vi "generate_plot.vi"(6 "High Voltage":sgl=2.0, 7 "Sens":dbl=12100000000000.0, 10 "Vnoise":dbl=0.005, 11 "Dust Array":T2[](array[typedef])=[{"Dust Event ID"=59, "Integer Timestamp"=1340138392671, "Velocity"=19145.19921875, "Mass"=9.709090342484041e-18, "Charge"=8.89689e-16, "Radius"=6.65219e-08, "Passed_3rd_Detector"=1, "High Voltage"=2.0, "+ High Voltage Supply"=0.0, "- High Voltage Supply"=0.0, "HV Control Difference"=0.0, "Vacuum Pressure"=0.0, "Radiation"=0.0, "Column Current"=0.0, "Lost Charge"=0.0, "Chain Current"=0.0, "Control High Voltage"=0.0, "Current Group Name:"="New Group Name", "Current Experiment Name:"="test", "Current Experiment Description:"="", "Estimate Source"=1, "Estimate Quality"=1, "File Location"=0, "Dust Type"="", "Dust Density"=0.0}, {"Dust Event ID"=61, "Integer Timestamp"=1340138406852, "Velocity"=9417.3203125, "Mass"=5.304340014877123e-17, "Charge"=1.17605e-15, "Radius"=1.17161e-07, "Passed_3rd_Detector"=1, "High Voltage"=2.0, "+ High Voltage Supply"=0.0, "- High Voltage Supply"=0.0, "HV Control Difference"=0.0, "Vacuum Pressure"=0.0, "Radiation"=0.0, "Column Current"=0.0, "Lost Charge"=0.0, "Chain Current"=0.0, "Control High Voltage"=0.0, "Current Group Name:"="New Group Name", "Current Experiment Name:"="test", "Current Experiment Description:"="", "Estimate Source"=1, "Estimate Quality"=1, "File Location"=0, "Dust Type"="", "Dust Density"=0.0}, {"Dust Event ID"=63, "Integer Timestamp"=1340138434737, "Velocity"=6076.06982421875, "Mass"=5.564189870760041e-17, "Charge"=5.13556e-16, "Radius"=1.19044e-07, "Passed_3rd_Detector"=1, "High Voltage"=2.0, "+ High Voltage Supply"=0.0, "- High Voltage Supply"=0.0, "HV Control Difference"=0.0, "Vacuum Pressure"=0.0, "Radiation"=0.0, "Column Current"=0.0, "Lost Charge"=0.0, "Chain Current"=0.0, "Control High Voltage"=0.0, "Current Group Name:"="New Group Name", "Current Experiment Name:"="test", "Current Experiment Description:"="", "Estimate Source"=1, "Estimate Quality"=1, "File Location"=0, "Dust Type"="", "Dust Density"=0.0}, {"Dust Event ID"=65, "Integer Timestamp"=1340138517545, "Velocity"=5796.47021484375, "Mass"=7.827660164472748e-16, "Charge"=6.57505e-15, "Radius"=2.87375e-07, "Passed_3rd_Detector"=1, "High Voltage"=2.0, "+ High Voltage Supply"=0.0, "- High Voltage Supply"=0.0, "HV Control Difference"=0.0, "Vacuum Pressure"=0.0, "Radiation"=0.0, "Column Current"=0.0, "Lost Charge"=0.0, "Chain Current"=0.0, "Control High Voltage"=0.0, "Current Group Name:"="New Group Name", "Current Experiment Name:"="test", "Current Experiment Description:"="", "Estimate Source"=1, "Estimate Quality"=1, "File Location"=0, "Dust Type"="", "Dust Density"=0.0}, {"Dust Event ID"=66, "Integer Timestamp"=1340138518480, "Velocity"=9192.0595703125, "Mass"=9.891599803709986e-17, "Charge"=2.08945e-15, "Radius"=1.4421e-07, "Passed_3rd_Detector"=1, "High Voltage"=2.0, "+ High Voltage Supply"=0.0, "- High Voltage Supply"=0.0, "HV Control Difference"=0.0, "Vacuum Pressure"=0.0, "Radiation"=0.0, "Column Current"=0.0, "Lost Charge"=0.0, "Chain Current"=0.0, "Control High Voltage"=0.0, "Current Group Name:"="New Group Name", "Current Experiment Name:"="test", "Current Experiment Description:"="", "Estimate Source"=1, "Estimate Quality"=1, "File Location"=0, "Dust Type"="", "Dust Density"=0.0}, {"Dust Event ID"=67, "Integer Timestamp"=1340138532228, "Velocity"=34719.30078125, "Mass"=2.6360200918000455e-18, "Charge"=7.94385e-16, "Radius"=4.30746e-08, "Passed_3rd_Detector"=1, "High Voltage"=2.0, "+ High Voltage Supply"=0.0, "- High Voltage Supply"=0.0, "HV Control Difference"=0.0, "Vacuum Pressure"=0.0, "Radiation"=0.0, "Column Current"=0.0, "Lost Charge"=0.0, "Chain Current"=0.0, "Control High Voltage"=0.0, "Current Group Name:"="New Group Name", "Current Experiment Name:"="test", "Current Experiment Description:"="", "Estimate Source"=1, "Estimate Quality"=1, "File Location"=0, "Dust Type"="", "Dust Density"=0.0}, {"Dust Event ID"=68, "Integer Timestamp"=1340138545545, "Velocity"=7001.97021484375, "Mass"=1.8855600591991987e-16, "Charge"=2.31111e-15, "Radius"=1.78807e-07, "Passed_3rd_Detector"=1, "High Voltage"=2.0, "+ High Voltage Supply"=0.0, "- High Voltage Supply"=0.0, "HV Control Difference"=0.0, "Vacuum Pressure"=0.0, "Radiation"=0.0, "Column Current"=0.0, "Lost Charge"=0.0, "Chain Current"=0.0, "Control High Voltage"=0.0, "Current Group Name:"="New Group Name", "Current Experiment Name:"="test", "Current Experiment Description:"="", "Estimate Source"=1, "Estimate Quality"=1, "File Location"=0, "Dust Type"="", "Dust Density"=0.0}, {"Dust Event ID"=73, "Integer Timestamp"=1340138752578, "Velocity"=19658.5, "Mass"=9.036869609983635e-18, "Charge"=8.7309e-16, "Radius"=6.49498e-08, "Passed_3rd_Detector"=1, "High Voltage"=2.0, "+ High Voltage Supply"=0.0, "- High Voltage Supply"=0.0, "HV Control Difference"=0.0, "Vacuum Pressure"=0.0, "Radiation"=0.0, "Column Current"=0.0, "Lost Charge"=0.0, "Chain Current"=0.0, "Control High Voltage"=0.0, "Current Group Name:"="New Group Name", "Current Experiment Name:"="test", "Current Experiment Description:"="", "Estimate Source"=1, "Estimate Quality"=1, "File Location"=0, "Dust Type"="", "Dust Density"=0.0}, {"Dust Event ID"=74, "Integer Timestamp"=1340138757697, "Velocity"=26103.69921875, "Mass"=5.479880065852002e-18, "Charge"=9.33502e-16, "Radius"=5.49746e-08, "Passed_3rd_Detector"=1, "High Voltage"=2.0, "+ High Voltage Supply"=0.0, "- High Voltage Supply"=0.0, "HV Control Difference"=0.0, "Vacuum Pressure"=0.0, "Radiation"=0.0, "Column Current"=0.0, "Lost Charge"=0.0, "Chain Current"=0.0, "Control High Voltage"=0.0, "Current Group Name:"="New Group Name", "Current Experiment Name:"="test", "Current Experiment Description:"="", "Estimate Source"=1, "Estimate Quality"=1, "File Location"=0, "Dust Type"="", "Dust Density"=0.0}, {"Dust Event ID"=75, "Integer Timestamp"=1340138762289, "Velocity"=11104.599609375, "Mass"=3.4991500151336583e-17, "Charge"=1.07872e-15, "Radius"=1.0199e-07, "Passed_3rd_Detector"=1, "High Voltage"=2.0, "+ High Voltage Supply"=0.0, "- High Voltage Supply"=0.0, "HV Control Difference"=0.0, "Vacuum Pressure"=0.0, "Radiation"=0.0, "Column Current"=0.0, "Lost Charge"=0.0, "Chain Current"=0.0, "Control High Voltage"=0.0, "Current Group Name:"="New Group Name", "Current Experiment Name:"="test", "Current Experiment Description:"="", "Estimate Source"=1, "Estimate Quality"=1, "File Location"=0, "Dust Type"="", "Dust Density"=0.0}, {"Dust Event ID"=76, "Integer Timestamp"=1340138792956, "Velocity"=7613.759765625, "Mass"=1.7990099679509583e-16, "Charge"=2.60719e-15, "Radius"=1.76029e-07, "Passed_3rd_Detector"=1, "High Voltage"=2.0, "+ High Voltage Supply"=0.0, "- High Voltage Supply"=0.0, "HV Control Difference"=0.0, "Vacuum Pressure"=0.0, "Radiation"=0.0, "Column Current"=0.0, "Lost Charge"=0.0, "Chain Current"=0.0, "Control High Voltage"=0.0, "Current Group Name:"="New Group Name", "Current Experiment Name:"="test", "Current Experiment Description:"="", "Estimate Source"=1, "Estimate Quality"=1, "File Location"=0, "Dust Type"="", "Dust Density"=0.0}, {"Dust Event ID"=80, "Integer Timestamp"=1340139107484, "Velocity"=34660.0, "Mass"=2.9206500454473984e-18, "Charge"=8.77155e-16, "Radius"=4.45723e-08, "Passed_3rd_Detector"=1, "High Voltage"=2.0, "+ High Voltage Supply"=0.0, "- High Voltage Supply"=0.0, "HV Control Difference"=0.0, "Vacuum Pressure"=0.0, "Radiation"=0.0, "Column Current"=0.0, "Lost Charge"=0.0, "Chain Current"=0.0, "Control High Voltage"=0.0, "Current Group Name:"="New Group Name", "Current Experiment Name:"="test", "Current Experiment Description:"="", "Estimate Source"=1, "Estimate Quality"=1, "File Location"=0, "Dust Type"="", "Dust Density"=0.0}, {"Dust Event ID"=85, "Integer Timestamp"=1340139269076, "Velocity"=7758.72021484375, "Mass"=1.2614399785804245e-16, "Charge"=1.89839e-15, "Radius"=1.56385e-07, "Passed_3rd_Detector"=1, "High Voltage"=2.0, "+ High Voltage Supply"=0.0, "- High Voltage Supply"=0.0, "HV Control Difference"=0.0, "Vacuum Pressure"=0.0, "Radiation"=0.0, "Column Current"=0.0, "Lost Charge"=0.0, "Chain Current"=0.0, "Control High Voltage"=0.0, "Current Group Name:"="New Group Name", "Current Experiment Name:"="test", "Current Experiment Description:"="", "Estimate Source"=1, "Estimate Quality"=1, "File Location"=0, "Dust Type"="", "Dust Density"=0.0}, {"Dust Event ID"=90, "Integer Timestamp"=1340139421851, "Velocity"=7551.02001953125, "Mass"=1.7357100046625623e-16, "Charge"=2.47417e-15, "Radius"=1.73939e-07, "Passed_3rd_Detector"=1, "High Voltage"=2.0, "+ High Voltage Supply"=0.0, "- High Voltage Supply"=0.0, "HV Control Difference"=0.0, "Vacuum Pressure"=0.0, "Radiation"=0.0, "Column Current"=0.0, "Lost Charge"=0.0, "Chain Current"=0.0, "Control High Voltage"=0.0, "Current Group Name:"="New Group Name", "Current Experiment Name:"="test", "Current Experiment Description:"="", "Estimate Source"=1, "Estimate Quality"=1, "File Location"=0, "Dust Type"="", "Dust Density"=0.0}, {"Dust Event ID"=92, "Integer Timestamp"=1340139600351, "Velocity"=17512.5, "Mass"=1.0332900329634781e-17, "Charge"=7.9224e-16, "Radius"=6.7917e-08, "Passed_3rd_Detector"=1, "High Voltage"=2.0, "+ High Voltage Supply"=0.0, "- High Voltage Supply"=0.0, "HV Control Difference"=0.0, "Vacuum Pressure"=0.0, "Radiation"=0.0, "Column Current"=0.0, "Lost Charge"=0.0, "Chain Current"=0.0, "Control High Voltage"=0.0, "Current Group Name:"="New Group Name", "Current Experiment Name:"="test", "Current Experiment Description:"="", "Estimate Source"=1, "Estimate Quality"=1, "File Location"=0, "Dust Type"="", "Dust Density"=0.0}, {"Dust Event ID"=95, "Integer Timestamp"=1340139724238, "Velocity"=28180.69921875, "Mass"=4.071129857718561e-18, "Charge"=8.08274e-16, "Radius"=4.97902e-08, "Passed_3rd_Detector"=1, "High Voltage"=2.0, "+ High Voltage Supply"=0.0, "- High Voltage Supply"=0.0, "HV Control Difference"=0.0, "Vacuum Pressure"=0.0, "Radiation"=0.0, "Column Current"=0.0, "Lost Charge"=0.0, "Chain Current"=0.0, "Control High Voltage"=0.0, "Current Group Name:"="New Group Name", "Current Experiment Name:"="test", "Current Experiment Description:"="", "Estimate Source"=1, "Estimate Quality"=1, "File Location"=0, "Dust Type"="", "Dust Density"=0.0}, {"Dust Event ID"=97, "Integer Timestamp"=1340139740652, "Velocity"=7861.9599609375, "Mass"=5.145899855115246e-17, "Charge"=7.95176e-16, "Radius"=1.15983e-07, "Passed_3rd_Detector"=1, "High Voltage"=2.0, "+ High Voltage Supply"=0.0, "- High Voltage Supply"=0.0, "HV Control Difference"=0.0, "Vacuum Pressure"=0.0, "Radiation"=0.0, "Column Current"=0.0, "Lost Charge"=0.0, "Chain Current"=0.0, "Control High Voltage"=0.0, "Current Group Name:"="New Group Name", "Current Experiment Name:"="test", "Current Experiment Description:"="", "Estimate Source"=1, "Estimate Quality"=1, "File Location"=0, "Dust Type"="", "Dust Density"=0.0}, {"Dust Event ID"=105, "Integer Timestamp"=1340140151192, "Velocity"=6723.72021484375, "Mass"=2.712949915359978e-16, "Charge"=3.0662e-15, "Radius"=2.01861e-07, "Passed_3rd_Detector"=1, "High Voltage"=2.0, "+ High Voltage Supply"=0.0, "- High Voltage Supply"=0.0, "HV Control Difference"=0.0, "Vacuum Pressure"=0.0, "Radiation"=0.0, "Column Current"=0.0, "Lost Charge"=0.0, "Chain Current"=0.0, "Control High Voltage"=0.0, "Current Group Name:"="New Group Name", "Current Experiment Name:"="test", "Current Experiment Description:"="", "Estimate Source"=1, "Estimate Quality"=1, "File Location"=0, "Dust Type"="", "Dust Density"=0.0}, {"Dust Event ID"=108, "Integer Timestamp"=1340140254486, "Velocity"=42754.19921875, "Mass"=1.9903799811034182e-18, "Charge"=9.09563e-16, "Radius"=3.92239e-08, "Passed_3rd_Detector"=1, "High Voltage"=2.0, "+ High Voltage Supply"=0.0, "- High Voltage Supply"=0.0, "HV Control Difference"=0.0, "Vacuum Pressure"=0.0, "Radiation"=0.0, "Column Current"=0.0, "Lost Charge"=0.0, "Chain Current"=0.0, "Control High Voltage"=0.0, "Current Group Name:"="New Group Name", "Current Experiment Name:"="test", "Current Experiment Description:"="", "Estimate Source"=1, "Estimate Quality"=1, "File Location"=0, "Dust Type"="", "Dust Density"=0.0}, {"Dust Event ID"=111, "Integer Timestamp"=1340140356251, "Velocity"=16529.599609375, "Mass"=1.0798100088689704e-17, "Charge"=7.37587e-16, "Radius"=6.89215e-08, "Passed_3rd_Detector"=1, "High Voltage"=2.0, "+ High Voltage Supply"=0.0, "- High Voltage Supply"=0.0, "HV Control Difference"=0.0, "Vacuum Pressure"=0.0, "Radiation"=0.0, "Column Current"=0.0, "Lost Charge"=0.0, "Chain Current"=0.0, "Control High Voltage"=0.0, "Current Group Name:"="New Group Name", "Current Experiment Name:"="test", "Current Experiment Description:"="", "Estimate Source"=1, "Estimate Quality"=1, "File Location"=0, "Dust Type"="", "Dust Density"=0.0}, {"Dust Event ID"=112, "Integer Timestamp"=1340140385957, "Velocity"=8983.150390625, "Mass"=9.722299755122023e-17, "Charge"=1.9614e-15, "Radius"=1.43382e-07, "Passed_3rd_Detector"=1, "High Voltage"=2.0, "+ High Voltage Supply"=0.0, "- High Voltage Supply"=0.0, "HV Control Difference"=0.0, "Vacuum Pressure"=0.0, "Radiation"=0.0, "Column Current"=0.0, "Lost Charge"=0.0, "Chain Current"=0.0, "Control High Voltage"=0.0, "Current Group Name:"="New Group Name", "Current Experiment Name:"="test", "Current Experiment Description:"="", "Estimate Source"=1, "Estimate Quality"=1, "File Location"=0, "Dust Type"="", "Dust Density"=0.0}, {"Dust Event ID"=113, "Integer Timestamp"=1340140387844, "Velocity"=29681.19921875, "Mass"=7.016149926141721e-17, "Charge"=1.54526e-14, "Radius"=1.28609e-07, "Passed_3rd_Detector"=1, "High Voltage"=2.0, "+ High Voltage Supply"=0.0, "- High Voltage Supply"=0.0, "HV Control Difference"=0.0, "Vacuum Pressure"=0.0, "Radiation"=0.0, "Column Current"=0.0, "Lost Charge"=0.0, "Chain Current"=0.0, "Control High Voltage"=0.0, "Current Group Name:"="New Group Name", "Current Experiment Name:"="test", "Current Experiment Description:"="", "Estimate Source"=1, "Estimate Quality"=1, "File Location"=0, "Dust Type"="", "Dust Density"=0.0}, {"Dust Event ID"=116, "Integer Timestamp"=1340140419545, "Velocity"=30761.19921875, "Mass"=4.625369819450529e-18, "Charge"=1.09419e-15, "Radius"=5.19542e-08, "Passed_3rd_Detector"=1, "High Voltage"=2.0, "+ High Voltage Supply"=0.0, "- High Voltage Supply"=0.0, "HV Control Difference"=0.0, "Vacuum Pressure"=0.0, "Radiation"=0.0, "Column Current"=0.0, "Lost Charge"=0.0, "Chain Current"=0.0, "Control High Voltage"=0.0, "Current Group Name:"="New Group Name", "Current Experiment Name:"="test", "Current Experiment Description:"="", "Estimate Source"=1, "Estimate Quality"=1, "File Location"=0, "Dust Type"="", "Dust Density"=0.0}, {"Dust Event ID"=118, "Integer Timestamp"=1340140449958, "Velocity"=23403.80078125, "Mass"=6.639849914495833e-18, "Charge"=9.09224e-16, "Radius"=5.86082e-08, "Passed_3rd_Detector"=1, "High Voltage"=2.0, "+ High Voltage Supply"=0.0, "- High Voltage Supply"=0.0, "HV Control Difference"=0.0, "Vacuum Pressure"=0.0, "Radiation"=0.0, "Column Current"=0.0, "Lost Charge"=0.0, "Chain Current"=0.0, "Control High Voltage"=0.0, "Current Group Name:"="New Group Name", "Current Experiment Name:"="test", "Current Experiment Description:"="", "Estimate Source"=1, "Estimate Quality"=1, "File Location"=0, "Dust Type"="", "Dust Density"=0.0}] {"File Location" items=["Unknown"=-1, "Storage"=0, "Processing"=1]; "Estimate Source" items=["Any Source."=-2, "No Shot"=-1, "Basic Labview Estimate"=0, "IDL Estimate From Andrew"=1, "IDL Estimate From Tobin"=2, "Old Metadata"=3]}) -> (3 "Dust Distribution":T1)   [LabVIEW 2013]
uses:
  User Interface/Controls/Query_Dust_Event.ctl
  User Interface/Controls/Estimate_source.ctl
  User Interface/Controls/File_location.ctl
  User Interface/Controls/Graph.ctl
  <userlib>/_OpenG.lib/array/array.llb/Search 1D Array (I8)__ogtk.vi
  <userlib>/_OpenG.lib/array/array.llb/Delete Elements from 2D Array (DBL)__ogtk.vi
panel:
  # "Dust Event"
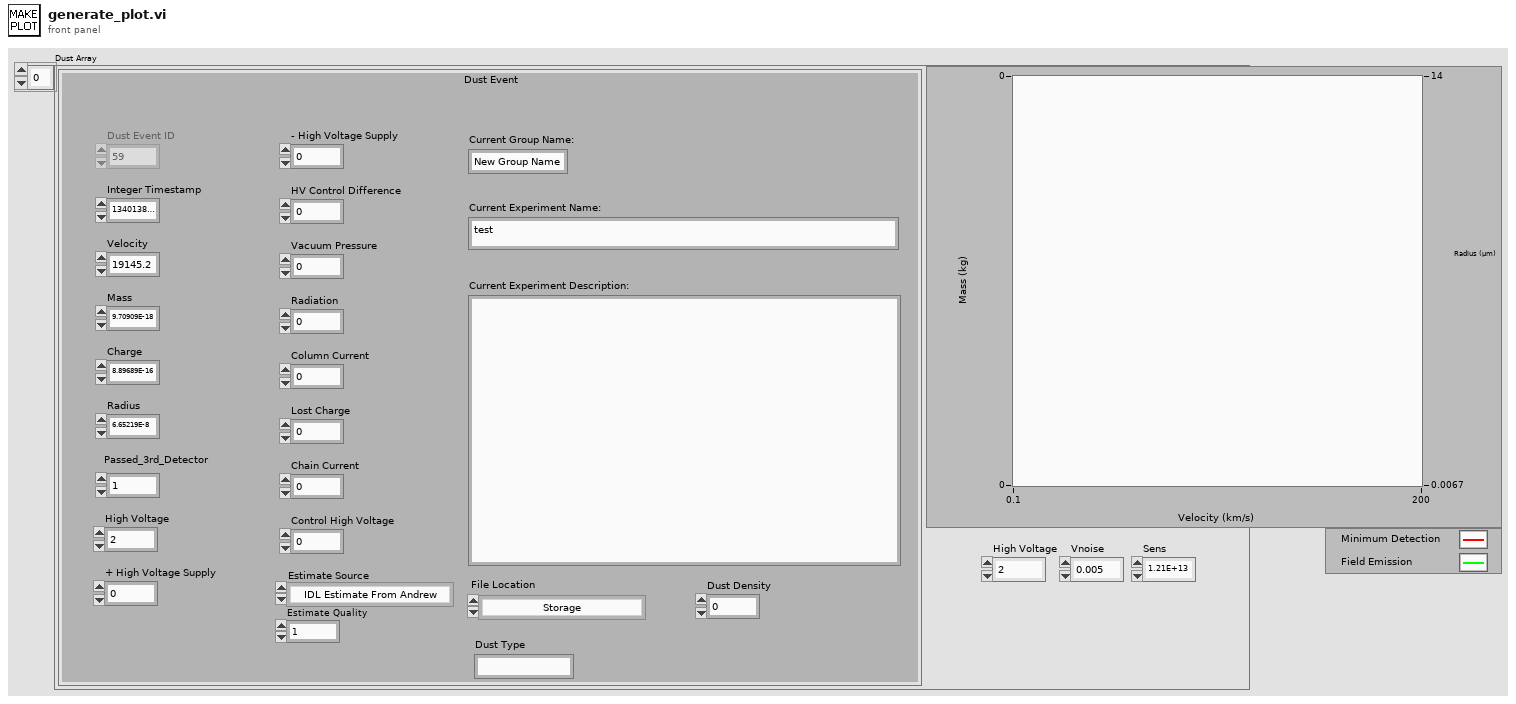
[diagram p1: front panel]
types:
  T1 = typedef "Graph.ctl" = cluster{cluster{"Vnoise":dbl, "Vnoise":dbl}[]}[]
  T2 = typedef "Query_Dust_Event.ctl" = cluster{"Dust Event ID":i64, "Integer Timestamp":i64, "Velocity":dbl, "Mass":dbl, "Charge":sgl, "Radius":sgl, "Passed_3rd_Detector":i8, "High Voltage":sgl, "+ High Voltage Supply":sgl, "- High Voltage Supply":sgl, "HV Control Difference":sgl, "Vacuum Pressure":sgl, "Radiation":sgl, "Column Current":sgl, "Lost Charge":sgl, "Chain Current":sgl, "Control High Voltage":sgl, "Current Group Name:":string, "Current Experiment Name:":string, "Current Experiment Description:":string, "Estimate Source":T3, "Estimate Quality":i8, "File Location":T4, "Dust Type":string, "Dust Density":sgl}
  T3 = typedef "Estimate_source.ctl" = i8
  T4 = typedef "File_location.ctl" = i8
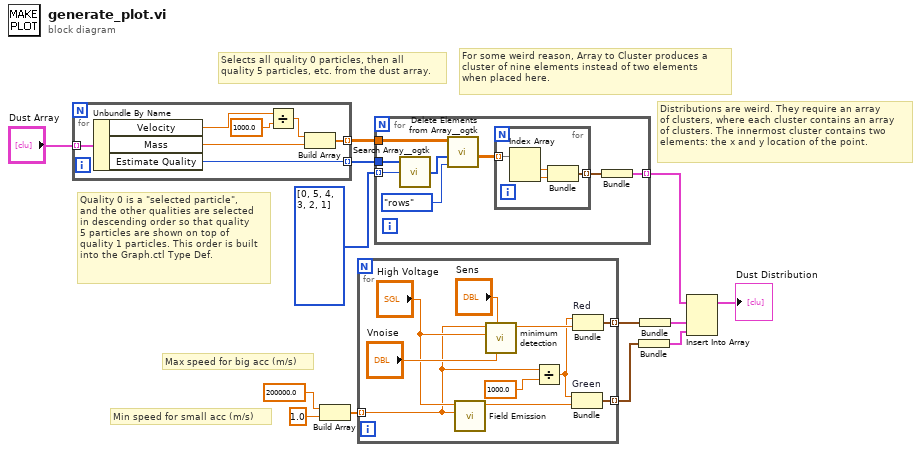
[diagram p0: block diagram]
diagram:
  # "Min speed for small acc (m/s)"
  # "Max speed for big acc (m/s)"
  # "Distributions are weird. They require an array\nof clusters, where each cluster contains an array\nof clusters. The innermost cluster contains two\nelements: the x and y location of the point."
  # "Selects all quality 0 particles, then all\nquality 5 particles, etc. from the dust array."
  # "For some weird reason, Array to Cluster produces a\ncluster of nine elements instead of two elements\nwhen placed here."
  # "Quality 0 is a \"selected particle\",\nand the other qualities are selected\nin descending order so that quality\n5 particles are shown on top of\nquality 1 particles. This order is built\ninto the Graph.ctl Type Def."
  n1 = for {
    tunnel: "Dust Array" -> [w20] mode=indexing
    tunnel: [w15] -> w4 mode=indexing
    tunnel: [w14] -> w3 mode=indexing
    n2 = Unbundle By Name(w20) -> ("Velocity"=w19:dbl, "Mass"=w16:dbl, "Estimate Quality"=w14:i8)
    n3 = Divide(x=w19, y=sgl 1000.0) -> (x/y=w17:dbl)
    n4 = Build Array(w17, w16) -> (w15:dbl[])
  }
  n5 = Build Array(sgl 200000.0 ("min value"), sgl 1.0 ("min value")) -> (w8:sgl[])
  n6 = for {
    tunnel: [w28] -> w13 mode=indexing
    tunnel: [w27] -> w12 mode=indexing
    tunnel: w8 -> [w22] mode=indexing
    n7 = call "Field Emission.vi"("Velocity"=w22, "Pelletron Volts"="High Voltage") -> ("Field Emission"=w26:ext)  [unwired: 9 in]
    n8 = call "minimum detection.vi"("Sens"="Sens", "Vnoise"="Vnoise", "Pelletron Volts"="High Voltage", "Velocity"=w22) -> ("Minimum Detection"=w25:dbl)  [unwired: 7 in]
    n9 = Divide(x=w22, y=sgl 1000.0) -> (x/y=w21:sgl)
    n10 = Bundle "Green"(w21, "Field Emission"=w26) -> (w27:cluster{sgl, "Field Emission":ext})  [unwired: 1 in]
    n11 = Bundle "Red"(w21, "Minimum Detection"=w25) -> (w28:cluster{sgl, "Minimum Detection":dbl})  [unwired: 1 in]
  }
  n12 = for {
    tunnel: w4 -> [w36]
    tunnel: w3 -> [w38]
    tunnel: i8[] [0, 5, 4, 3, 2, 1] -> [w37] mode=indexing
    tunnel: [w31] -> w1 mode=indexing
    n13 = call-poly <userlib>:"Search Array__ogtk.vi"("Array"=w38, "Element Data"=w37) -> ("Indices of Elements"=w34:i32[])  [unwired: 7 in]
    n14 = call-poly <userlib>:"Delete Elements from Array__ogtk.vi"("delete (rows or columns)"=enum16{"rows", "columns"}."rows", "indices"=w34, "array"=w36) -> ("deleted elements"=w33:dbl[][])  [unwired: 7 in, 1 out]
    n15 = for {
      tunnel: w33 -> [w42] mode=indexing
      tunnel: [w39] -> w32 mode=indexing
      n16 = Index Array(array=w42) -> (element #1=w40:dbl, element #2=w41:dbl)  [unwired: 2 in]
      n17 = Bundle(w40, w41) -> (w39:cluster{dbl, dbl})  [unwired: 1 in]
    }
    n18 = Bundle(w32) -> (w31:cluster{cluster{dbl, dbl}[]})  [unwired: 1 in]
  }
  n19 = Bundle ("Green")(w12) -> (w6:cluster{cluster{sgl, "Field Emission":ext}[]})  [unwired: 1 in]
  n20 = Bundle ("Red")(w13) -> (w7:cluster{cluster{sgl, "Minimum Detection":dbl}[]})  [unwired: 1 in]
  n21 = Insert Into Array(array=w1, new element #1=w7, new element #2=w6) -> (→"Dust Distribution":cluster{cluster{dbl, dbl}[]}[])  [unwired: 1 in]
